vi "Oqus GUID Lookup.vi"() -> ()   [LabVIEW 2014, in "Oqus Custom Device.lvlib"]
doc: "Use this Global VI to access the GUIDs assigned to the page resources of the Custom Device."
uses:
  Oqus Custom Device.lvlib
panel:
  in  "Custom Device":string="35f2e757-0c29-4d89-97e9-6f9421cf693d"
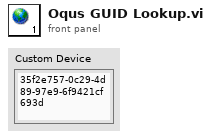
[diagram p1: front panel]
diagram:
